vi "メイン.vi"() -> (2 "測定周期/ms":dbl, 3 "値転記用配列":T2[](array[typedef]))   [LabVIEW 2021] (continued)
                          n3108 = Add(x=w5491, y=10) -> (x+y=w5482:i32)
                          n3109 = local read "csv作成表"() -> (w5478:string[][])
                          n3110 = Unbundle By Name(w5489) -> ("実測値(MAX)"=w5485:string, "実測値(MIN)"=w5486:string)
                          n3111 = Replace Array Subset(array=w5478, new element #1=w5485, index (row) #1=w5483, index (col) #1=w5484, new element #2=w5486, index (row) #2=w5483, index (col) #2=w5482) -> (w5480:string[][])
                          n3112 = Select(t=w5480, s=w5490, f=w5478) -> (s? t:f=w5481:string[][])
                          n3113 = local write "csv作成表"(w5481) -> ()
                        }
                        frame 8 {
                          w5501 = 2
                          # "B"
                          # "A"
                          # "csv作成の為表へクラスタ(実測値)書き込み"
                          # "⑤"
                          # "③"
                          # "④"
                          n3114 = local read "メインON/OFF_\n設定 9"() -> (w5512:T1)
                          n3115 = Unbundle By Name(w5512) -> ("使用ON/OFF"=w5508:bool)
                          n3116 = control-ref of="前回値転記用配列"() -> (w5506:refnum<vi>)
                          n3117 = local read "メイン設定_設定 9"() -> (w5513:T2)
                          n3118 = call "メイン_測定値配列_CSV転記サブ.vi"("メイン設定_設定入力"=w5513, "ループ反復数値入力"=w5510, "実測設定項目"=w5511, "使用ON/OFF"=w5508, "前回値転記用配列"=w5506) -> ("ループ反復数値出力"=w5509:i32, "メイン設定_設定出力"=w5507:T2)  [unwired: 5 in]
                          n3119 = local write "メイン設定_設定 9"(w5507) -> ()
                          n3120 = Add(x=10, y=w5509) -> (x+y=w5502:i32)
                          n3121 = Add(x=w5509, y=11) -> (x+y=w5500:i32)
                          n3122 = local read "csv作成表"() -> (w5496:string[][])
                          n3123 = Unbundle By Name(w5507) -> ("実測値(MAX)"=w5503:string, "実測値(MIN)"=w5504:string)
                          n3124 = Replace Array Subset(array=w5496, new element #1=w5503, index (row) #1=w5501, index (col) #1=w5502, new element #2=w5504, index (row) #2=w5501, index (col) #2=w5500) -> (w5498:string[][])
                          n3125 = Select(t=w5498, s=w5508, f=w5496) -> (s? t:f=w5499:string[][])
                          n3126 = local write "csv作成表"(w5499) -> ()
                        }
                        frame 9 {
                          w5519 = 2
                          # "B"
                          # "A"
                          # "csv作成の為表へクラスタ(実測値)書き込み"
                          # "⑤"
                          # "③"
                          # "④"
                          n3127 = local read "メインON/OFF_\n設定 10"() -> (w5530:T1)
                          n3128 = Unbundle By Name(w5530) -> ("使用ON/OFF"=w5526:bool)
                          n3129 = control-ref of="前回値転記用配列"() -> (w5524:refnum<vi>)
                          n3130 = local read "メイン設定_設定 10"() -> (w5531:T2)
                          n3131 = call "メイン_測定値配列_CSV転記サブ.vi"("メイン設定_設定入力"=w5531, "ループ反復数値入力"=w5528, "実測設定項目"=w5529, "使用ON/OFF"=w5526, "前回値転記用配列"=w5524) -> ("ループ反復数値出力"=w5527:i32, "メイン設定_設定出力"=w5525:T2)  [unwired: 5 in]
                          n3132 = local write "メイン設定_設定 10"(w5525) -> ()
                          n3133 = Add(x=11, y=w5527) -> (x+y=w5520:i32)
                          n3134 = Add(x=w5527, y=12) -> (x+y=w5518:i32)
                          n3135 = local read "csv作成表"() -> (w5514:string[][])
                          n3136 = Unbundle By Name(w5525) -> ("実測値(MAX)"=w5521:string, "実測値(MIN)"=w5522:string)
                          n3137 = Replace Array Subset(array=w5514, new element #1=w5521, index (row) #1=w5519, index (col) #1=w5520, new element #2=w5522, index (row) #2=w5519, index (col) #2=w5518) -> (w5516:string[][])
                          n3138 = Select(t=w5516, s=w5526, f=w5514) -> (s? t:f=w5517:string[][])
                          n3139 = local write "csv作成表"(w5517) -> ()
                        }
                        frame 10 {
                          w5537 = 2
                          # "B"
                          # "A"
                          # "csv作成の為表へクラスタ(実測値)書き込み"
                          # "⑤"
                          # "③"
                          # "④"
                          n3140 = local read "メインON/OFF_\n設定 11"() -> (w5548:T1)
                          n3141 = Unbundle By Name(w5548) -> ("使用ON/OFF"=w5544:bool)
                          n3142 = control-ref of="前回値転記用配列"() -> (w5542:refnum<vi>)
                          n3143 = local read "メイン設定_設定 11"() -> (w5549:T2)
                          n3144 = call "メイン_測定値配列_CSV転記サブ.vi"("メイン設定_設定入力"=w5549, "ループ反復数値入力"=w5546, "実測設定項目"=w5547, "使用ON/OFF"=w5544, "前回値転記用配列"=w5542) -> ("ループ反復数値出力"=w5545:i32, "メイン設定_設定出力"=w5543:T2)  [unwired: 5 in]
                          n3145 = local write "メイン設定_設定 11"(w5543) -> ()
                          n3146 = Add(x=12, y=w5545) -> (x+y=w5538:i32)
                          n3147 = Add(x=w5545, y=13) -> (x+y=w5536:i32)
                          n3148 = local read "csv作成表"() -> (w5532:string[][])
                          n3149 = Unbundle By Name(w5543) -> ("実測値(MAX)"=w5539:string, "実測値(MIN)"=w5540:string)
                          n3150 = Replace Array Subset(array=w5532, new element #1=w5539, index (row) #1=w5537, index (col) #1=w5538, new element #2=w5540, index (row) #2=w5537, index (col) #2=w5536) -> (w5534:string[][])
                          n3151 = Select(t=w5534, s=w5544, f=w5532) -> (s? t:f=w5535:string[][])
                          n3152 = local write "csv作成表"(w5535) -> ()
                        }
                        frame 11 {
                          w5555 = 2
                          # "B"
                          # "A"
                          # "csv作成の為表へクラスタ(実測値)書き込み"
                          # "⑤"
                          # "③"
                          # "④"
                          n3153 = local read "メインON/OFF_\n設定 12"() -> (w5566:T1)
                          n3154 = Unbundle By Name(w5566) -> ("使用ON/OFF"=w5562:bool)
                          n3155 = control-ref of="前回値転記用配列"() -> (w5560:refnum<vi>)
                          n3156 = local read "メイン設定_設定 12"() -> (w5567:T2)
                          n3157 = call "メイン_測定値配列_CSV転記サブ.vi"("メイン設定_設定入力"=w5567, "ループ反復数値入力"=w5564, "実測設定項目"=w5565, "使用ON/OFF"=w5562, "前回値転記用配列"=w5560) -> ("ループ反復数値出力"=w5563:i32, "メイン設定_設定出力"=w5561:T2)  [unwired: 5 in]
                          n3158 = local write "メイン設定_設定 12"(w5561) -> ()
                          n3159 = Add(x=13, y=w5563) -> (x+y=w5556:i32)
                          n3160 = Add(x=w5563, y=14) -> (x+y=w5554:i32)
                          n3161 = local read "csv作成表"() -> (w5550:string[][])
                          n3162 = Unbundle By Name(w5561) -> ("実測値(MAX)"=w5557:string, "実測値(MIN)"=w5558:string)
                          n3163 = Replace Array Subset(array=w5550, new element #1=w5557, index (row) #1=w5555, index (col) #1=w5556, new element #2=w5558, index (row) #2=w5555, index (col) #2=w5554) -> (w5552:string[][])
                          n3164 = Select(t=w5552, s=w5562, f=w5550) -> (s? t:f=w5553:string[][])
                          n3165 = local write "csv作成表"(w5553) -> ()
                        }
                      }
                    }
                  }
                }
                n3166 = local write "値転記用配列"(w5324) -> ()
                n3167 = flat-sequence {
                  tunnel: [w5339] -> w5325
                  tunnel: w5324 -> [w5339]
                  frame #0 {
                    w5334 = T9 {"Horizontal"=-51, "Vertical"=504} ("座標 7")
                    n3168 = control-ref of="このVI"() -> (w5335:refnum<vi>)
                    n3169 = property on="ペーン 2" class="Pane"("Origin"=w5334) -> ()  [unwired: 2 in, 2 out]
                    n3170 = property on="ペーン 2" class="Pane"("Origin"=w5334) -> ()  [unwired: 2 in, 2 out]
                    n3171 = control-ref of="このVI"() -> (w5337:refnum<vi>)
                    n3172 = Unbundle(w5334) -> ("Vertical"=w5336:i16)  [unwired: 1 out]
                    n3173 = Unbundle(w5334) -> ("Vertical"=w5338:i16)  [unwired: 1 out]
                    n3174 = call "メイン_装飾移動サブ.vi"("Y軸座標入力"=w5336, "VI入力"=w5335) -> ()  [unwired: 10 in]
                    n3175 = call "メイン_装飾枠移動サブ.vi"("Y軸座標入力"=w5338, "VI入力"=w5337) -> ()  [unwired: 10 in]
                  }
                }
              }
              frame #1 {
                w5569 = T8."Enabled" ("無効")
                # "⑪ボタンの無効解除"
                n3176 = local write "測定新値\nリセット用 8"(TRUE) -> ()
                n3177 = for {
                  N: 12 -> [_]
                  tunnel: w5569 -> [w5572]
                  i -> [w5573]
                  n3178 = case shown="11" w5573 {
                    tunnel: w5572 -> [w5574 w5575 w5576 w5577 w5578 w5579 w5580 w5581 w5582 w5583 w5584 w5585]
                    frame 0, Default {
                      n3179 = property on="メイン測定ボタン_単発 1" class="Bool (指定)"("DisabledEnum"=w5574) -> ()  [unwired: 2 in, 2 out]
                      n3180 = property on="メイン測定ボタン_連続 1" class="Bool (指定)"("DisabledEnum"=w5574) -> ()  [unwired: 2 in, 2 out]
                    }
                    frame 1 {
                      n3181 = property on="メイン測定ボタン_単発 2" class="Bool (指定)"("DisabledEnum"=w5575) -> ()  [unwired: 2 in, 2 out]
                      n3182 = property on="メイン測定ボタン_連続 2" class="Bool (指定)"("DisabledEnum"=w5575) -> ()  [unwired: 2 in, 2 out]
                    }
                    frame 2 {
                      n3183 = property on="メイン測定ボタン_単発 3" class="Bool (指定)"("DisabledEnum"=w5576) -> ()  [unwired: 2 in, 2 out]
                      n3184 = property on="メイン測定ボタン_連続 3" class="Bool (指定)"("DisabledEnum"=w5576) -> ()  [unwired: 2 in, 2 out]
                    }
                    frame 3 {
                      n3185 = property on="メイン測定ボタン_単発 4" class="Bool (指定)"("DisabledEnum"=w5577) -> ()  [unwired: 2 in, 2 out]
                      n3186 = property on="メイン測定ボタン_連続 4" class="Bool (指定)"("DisabledEnum"=w5577) -> ()  [unwired: 2 in, 2 out]
                    }
                    frame 4 {
                      n3187 = property on="メイン測定ボタン_単発 5" class="Bool (指定)"("DisabledEnum"=w5578) -> ()  [unwired: 2 in, 2 out]
                      n3188 = property on="メイン測定ボタン_連続 5" class="Bool (指定)"("DisabledEnum"=w5578) -> ()  [unwired: 2 in, 2 out]
                    }
                    frame 5 {
                      n3189 = property on="メイン測定ボタン_連続 6" class="Bool (指定)"("DisabledEnum"=w5579) -> ()  [unwired: 2 in, 2 out]
                      n3190 = property on="メイン測定ボタン_単発 6" class="Bool (指定)"("DisabledEnum"=w5579) -> ()  [unwired: 2 in, 2 out]
                    }
                    frame 6 {
                      n3191 = property on="メイン測定ボタン_連続 7" class="Bool (指定)"("DisabledEnum"=w5580) -> ()  [unwired: 2 in, 2 out]
                      n3192 = property on="メイン測定ボタン_単発 7" class="Bool (指定)"("DisabledEnum"=w5580) -> ()  [unwired: 2 in, 2 out]
                    }
                    frame 7 {
                      n3193 = property on="メイン測定ボタン_単発 8" class="Bool (指定)"("DisabledEnum"=w5581) -> ()  [unwired: 2 in, 2 out]
                      n3194 = property on="メイン測定ボタン_連続 8" class="Bool (指定)"("DisabledEnum"=w5581) -> ()  [unwired: 2 in, 2 out]
                    }
                    frame 8 {
                      n3195 = property on="メイン測定ボタン_単発 9" class="Bool (指定)"("DisabledEnum"=w5582) -> ()  [unwired: 2 in, 2 out]
                      n3196 = property on="メイン測定ボタン_連続 9" class="Bool (指定)"("DisabledEnum"=w5582) -> ()  [unwired: 2 in, 2 out]
                    }
                    frame 9 {
                      n3197 = property on="メイン測定ボタン_単発 10" class="Bool (指定)"("DisabledEnum"=w5583) -> ()  [unwired: 2 in, 2 out]
                      n3198 = property on="メイン測定ボタン_連続 10" class="Bool (指定)"("DisabledEnum"=w5583) -> ()  [unwired: 2 in, 2 out]
                    }
                    frame 10 {
                      n3199 = property on="メイン測定ボタン_単発 11" class="Bool (指定)"("DisabledEnum"=w5584) -> ()  [unwired: 2 in, 2 out]
                      n3200 = property on="メイン測定ボタン_連続 11" class="Bool (指定)"("DisabledEnum"=w5584) -> ()  [unwired: 2 in, 2 out]
                    }
                    frame 11 {
                      n3201 = property on="メイン測定ボタン_連続 12" class="Bool (指定)"("DisabledEnum"=w5585) -> ()  [unwired: 2 in, 2 out]
                      n3202 = property on="メイン測定ボタン_単発 12" class="Bool (指定)"("DisabledEnum"=w5585) -> ()  [unwired: 2 in, 2 out]
                    }
                  }
                }
                n3203 = property on="TOPページへ" class="Bool"("DisabledEnum"=w5569) -> ()  [unwired: 2 in, 2 out]
                n3204 = property on="保存して終了" class="Bool"("DisabledEnum"=w5569) -> ()  [unwired: 2 in, 2 out]
                n3205 = property on="保存せずに" class="Bool"("DisabledEnum"=w5569) -> ()  [unwired: 2 in, 2 out]
              }
            }
          }
          frame True {
          }
        }
      }
      frame "測定9" {
        # "⑦"
        # "項目別のボタンで測定を行う為、項目分必要"
        n3206 = local read "測定旧値 9"() -> (w5589:bool)
        n3207 = case shown="FALSE" w5589 {
          tunnel: w5587 -> [w5592 w5855]
          tunnel: [w5591 w5855] -> w5588
          frame False {
            n3208 = flat-sequence {
              tunnel: w5592 -> [w5602]
              tunnel: [w5594] -> w5590
              tunnel: [w5840] -> w5591
              tunnel: w5590 -> [w5840]
              frame #0 {
                # "※複製コピー時変更する項目\n①②\nローカル変数\n\n入れ子のケースストラクチャ\"2\"を複製\n\n0～数だけ変更する\n③④⑤\nローカル変数\n\n※AB\n行番号の変更をする必要がある\n\n--------------------------------\nこの後イベントストラクチャ複製する\n--------------------------------\nイベントストラクチャ複製後\n\n⑦⑧\nローカル変数\n⑨\n装飾体の位置設定\n-51は固定\n前ケースの数値+72\n⑩\n測定新値リセット用\nのボタンが複製されているので、\nフロントパネルを整理する\n⑪\nプロパティノード\nボタンの無効解除クリア以外全てのボタン対象"
                # "実測完了の簡易疑似コード\n\n1)測定モードが単発・連続、多点かで転記する配列を変える\n2)値転記用配列へ転記\n\nここからゲージ分を繰り返す必要がある\n\n3)配列0を取り出す\n4)配列0のポートNoを取り出す\n5)メイン測定_設定配列(測定1の対象配列)のポートNoと比較\n6)同じだったら処理をする。違ったら何もしない\n7)同じだったら配列0のメインON/OFF_設定1の使用ON/OFFがTrueかFalseか\nFlaseだったら前回値転記用配列から前回の値をメイン設定_設定へ転記\nTrueだったらメイン設定_設定の測定モードから\n0単発、1連続、3多点\nの処理を行う\n8)測定値をメイン設定_設定へ転記したら、前回転記用配列へ転記する"
                # "⑨"
                # "⑧"
                # "②"
                # "グループNO(表示上はポートNo)が同じだったら値を転記する\n\n測定した配列のグループNOと値転記用配列の他の指標グループNOを比較する\n＝だったら、対象の配列のON/OFFボタンがTrueか確認し、\nTrueだったら、測定モードによって、値かMAX、MINの数値を転記する\n\nグループNOが同じでなければ、転記しない(何もしない)"
                # "まず値転記用配列に測定の値を転記"
                # "実測定画面vi動作"
                n3209 = local read "メイン設定_設定 9"() -> (w5597:T2)
                n3210 = local read "測定新値 9"() -> (→"測定新値\nリセット用 9":bool)
                n3211 = local read "測定周期/ms"() -> (w5595:dbl)
                n3212 = Unbundle By Name(w5597) -> ("測定モード"=w5598:u16)
                n3213 = call "実測定画面.vi"("実測設定項目配列_\nメインからの転記"=w5602, "測定周期/ms_制御器"=w5595) -> ("実測設定項目配列_\nゲージIOへ転記用"=w5600:T2[], "実測設定項目配列_\n多点測定メイン転記用"=w5599:T2[])  [unwired: 11 in, 1 out]
                n3214 = case shown="1" w5598 {
                  tunnel: w5600 -> [w5609 w5610 _]
                  tunnel: [w5609 w5610 w5611] -> w5593
                  tunnel: w5599 -> [_ _ w5611]
                  frame 0, Default {
                  }
                  frame 1 {
                  }
                  frame 2 {
                  }
                }
                n3215 = for {
                  N: 32 -> [_]
                  tunnel: w5593 -> [w5618]
                  i -> [w5613]
                  # "①"
                  # "※複製コピーはこのケースで行う"
                  # "32回分"
                  # "比較する固定GNO"
                  n3216 = local read "メイン設定_設定 9"() -> (w5612:T2)
                  n3217 = Index Array(array=w5618, index=w5613) -> (element=w5617:T2)
                  n3218 = Unbundle By Name(w5612) -> ("ポートNo."=w5616:dbl)
                  n3219 = Unbundle By Name(w5617) -> ("ポートNo."=w5615:dbl)
                  n3220 = Equal?(x=w5616, y=w5615) -> (x = y?=w5614:bool)
                  n3221 = case shown="TRUE" w5614 {
                    tunnel: w5617 -> [_ w5620]
                    tunnel: w5613 -> [_ w5619]
                    frame False {
                    }
                    frame True {
                      n3222 = case shown="0, デフォルト" w5619 {
                        tunnel: w5620 -> [w5636 w5654 w5672 w5690 w5708 w5726 w5744 w5762 w5780 w5798 w5816 w5834]
                        tunnel: w5619 -> [w5635 w5653 w5671 w5689 w5707 w5725 w5743 w5761 w5779 w5797 w5815 w5833]
                        frame 0, Default {
                          w5626 = 2
                          # "B"
                          # "A"
                          # "csv作成の為表へクラスタ(実測値)書き込み"
                          # "⑤"
                          # "③"
                          # "④"
                          n3223 = local read "メインON/OFF_\n設定 1"() -> (w5637:T1)
                          n3224 = Unbundle By Name(w5637) -> ("使用ON/OFF"=w5633:bool)
                          n3225 = control-ref of="前回値転記用配列"() -> (w5631:refnum<vi>)
                          n3226 = local read "メイン設定_設定 1"() -> (w5638:T2)
                          n3227 = call "メイン_測定値配列_CSV転記サブ.vi"("メイン設定_設定入力"=w5638, "ループ反復数値入力"=w5635, "実測設定項目"=w5636, "使用ON/OFF"=w5633, "前回値転記用配列"=w5631) -> ("ループ反復数値出力"=w5634:i32, "メイン設定_設定出力"=w5632:T2)  [unwired: 5 in]
                          n3228 = local write "メイン設定_設定 1"(w5632) -> ()
                          n3229 = Add(x=2, y=w5634) -> (x+y=w5627:i32)
                          n3230 = Add(x=w5634, y=3) -> (x+y=w5625:i32)
                          n3231 = local read "csv作成表"() -> (w5621:string[][])
                          n3232 = Unbundle By Name(w5632) -> ("実測値(MAX)"=w5628:string, "実測値(MIN)"=w5629:string)
                          n3233 = Replace Array Subset(array=w5621, new element #1=w5628, index (row) #1=w5626, index (col) #1=w5627, new element #2=w5629, index (row) #2=w5626, index (col) #2=w5625) -> (w5623:string[][])
                          n3234 = Select(t=w5623, s=w5633, f=w5621) -> (s? t:f=w5624:string[][])
                          n3235 = local write "csv作成表"(w5624) -> ()
                        }
                        frame 1 {
                          w5644 = 2
                          # "B"
                          # "A"
                          # "csv作成の為表へクラスタ(実測値)書き込み"
                          # "⑤"
                          # "③"
                          # "④"
                          n3236 = local read "メインON/OFF_\n設定 2"() -> (w5655:T1)
                          n3237 = Unbundle By Name(w5655) -> ("使用ON/OFF"=w5651:bool)
                          n3238 = control-ref of="前回値転記用配列"() -> (w5649:refnum<vi>)
                          n3239 = local read "メイン設定_設定 2"() -> (w5656:T2)
                          n3240 = call "メイン_測定値配列_CSV転記サブ.vi"("メイン設定_設定入力"=w5656, "ループ反復数値入力"=w5653, "実測設定項目"=w5654, "使用ON/OFF"=w5651, "前回値転記用配列"=w5649) -> ("ループ反復数値出力"=w5652:i32, "メイン設定_設定出力"=w5650:T2)  [unwired: 5 in]
                          n3241 = local write "メイン設定_設定 2"(w5650) -> ()
                          n3242 = Add(x=3, y=w5652) -> (x+y=w5645:i32)
                          n3243 = Add(x=w5652, y=4) -> (x+y=w5643:i32)
                          n3244 = local read "csv作成表"() -> (w5639:string[][])
                          n3245 = Unbundle By Name(w5650) -> ("実測値(MAX)"=w5646:string, "実測値(MIN)"=w5647:string)
                          n3246 = Replace Array Subset(array=w5639, new element #1=w5646, index (row) #1=w5644, index (col) #1=w5645, new element #2=w5647, index (row) #2=w5644, index (col) #2=w5643) -> (w5641:string[][])
                          n3247 = Select(t=w5641, s=w5651, f=w5639) -> (s? t:f=w5642:string[][])
                          n3248 = local write "csv作成表"(w5642) -> ()
                        }
                        frame 2 {
                          w5662 = 2
                          # "B"
                          # "A"
                          # "csv作成の為表へクラスタ(実測値)書き込み"
                          # "⑤"
                          # "③"
                          # "④"
                          n3249 = local read "メインON/OFF_\n設定 3"() -> (w5673:T1)
                          n3250 = Unbundle By Name(w5673) -> ("使用ON/OFF"=w5669:bool)
                          n3251 = control-ref of="前回値転記用配列"() -> (w5667:refnum<vi>)
                          n3252 = local read "メイン設定_設定 3"() -> (w5674:T2)
                          n3253 = call "メイン_測定値配列_CSV転記サブ.vi"("メイン設定_設定入力"=w5674, "ループ反復数値入力"=w5671, "実測設定項目"=w5672, "使用ON/OFF"=w5669, "前回値転記用配列"=w5667) -> ("ループ反復数値出力"=w5670:i32, "メイン設定_設定出力"=w5668:T2)  [unwired: 5 in]
                          n3254 = local write "メイン設定_設定 3"(w5668) -> ()
                          n3255 = Add(x=4, y=w5670) -> (x+y=w5663:i32)
                          n3256 = Add(x=w5670, y=5) -> (x+y=w5661:i32)
                          n3257 = local read "csv作成表"() -> (w5657:string[][])
                          n3258 = Unbundle By Name(w5668) -> ("実測値(MAX)"=w5664:string, "実測値(MIN)"=w5665:string)
                          n3259 = Replace Array Subset(array=w5657, new element #1=w5664, index (row) #1=w5662, index (col) #1=w5663, new element #2=w5665, index (row) #2=w5662, index (col) #2=w5661) -> (w5659:string[][])
                          n3260 = Select(t=w5659, s=w5669, f=w5657) -> (s? t:f=w5660:string[][])
                          n3261 = local write "csv作成表"(w5660) -> ()
                        }
                        frame 3 {
                          w5680 = 2
                          # "B"
                          # "A"
                          # "csv作成の為表へクラスタ(実測値)書き込み"
                          # "⑤"
                          # "③"
                          # "④"
                          n3262 = local read "メインON/OFF_\n設定 4"() -> (w5691:T1)
                          n3263 = Unbundle By Name(w5691) -> ("使用ON/OFF"=w5687:bool)
                          n3264 = control-ref of="前回値転記用配列"() -> (w5685:refnum<vi>)
                          n3265 = local read "メイン設定_設定 4"() -> (w5692:T2)
                          n3266 = call "メイン_測定値配列_CSV転記サブ.vi"("メイン設定_設定入力"=w5692, "ループ反復数値入力"=w5689, "実測設定項目"=w5690, "使用ON/OFF"=w5687, "前回値転記用配列"=w5685) -> ("ループ反復数値出力"=w5688:i32, "メイン設定_設定出力"=w5686:T2)  [unwired: 5 in]
                          n3267 = local write "メイン設定_設定 4"(w5686) -> ()
                          n3268 = Add(x=5, y=w5688) -> (x+y=w5681:i32)
                          n3269 = Add(x=w5688, y=6) -> (x+y=w5679:i32)
                          n3270 = local read "csv作成表"() -> (w5675:string[][])
                          n3271 = Unbundle By Name(w5686) -> ("実測値(MAX)"=w5682:string, "実測値(MIN)"=w5683:string)
                          n3272 = Replace Array Subset(array=w5675, new element #1=w5682, index (row) #1=w5680, index (col) #1=w5681, new element #2=w5683, index (row) #2=w5680, index (col) #2=w5679) -> (w5677:string[][])
                          n3273 = Select(t=w5677, s=w5687, f=w5675) -> (s? t:f=w5678:string[][])
                          n3274 = local write "csv作成表"(w5678) -> ()
                        }
                        frame 4 {
                          w5698 = 2
                          # "B"
                          # "A"
                          # "csv作成の為表へクラスタ(実測値)書き込み"
                          # "⑤"
                          # "③"
                          # "④"
                          n3275 = local read "メインON/OFF_\n設定 5"() -> (w5709:T1)
                          n3276 = Unbundle By Name(w5709) -> ("使用ON/OFF"=w5705:bool)
                          n3277 = control-ref of="前回値転記用配列"() -> (w5703:refnum<vi>)
                          n3278 = local read "メイン設定_設定 5"() -> (w5710:T2)
                          n3279 = call "メイン_測定値配列_CSV転記サブ.vi"("メイン設定_設定入力"=w5710, "ループ反復数値入力"=w5707, "実測設定項目"=w5708, "使用ON/OFF"=w5705, "前回値転記用配列"=w5703) -> ("ループ反復数値出力"=w5706:i32, "メイン設定_設定出力"=w5704:T2)  [unwired: 5 in]
                          n3280 = local write "メイン設定_設定 5"(w5704) -> ()
                          n3281 = Add(x=6, y=w5706) -> (x+y=w5699:i32)
                          n3282 = Add(x=w5706, y=7) -> (x+y=w5697:i32)
                          n3283 = local read "csv作成表"() -> (w5693:string[][])
                          n3284 = Unbundle By Name(w5704) -> ("実測値(MAX)"=w5700:string, "実測値(MIN)"=w5701:string)
                          n3285 = Replace Array Subset(array=w5693, new element #1=w5700, index (row) #1=w5698, index (col) #1=w5699, new element #2=w5701, index (row) #2=w5698, index (col) #2=w5697) -> (w5695:string[][])
                          n3286 = Select(t=w5695, s=w5705, f=w5693) -> (s? t:f=w5696:string[][])
                          n3287 = local write "csv作成表"(w5696) -> ()
                        }
                        frame 5 {
                          w5716 = 2
                          # "B"
                          # "A"
                          # "csv作成の為表へクラスタ(実測値)書き込み"
                          # "⑤"
                          # "③"
                          # "④"
                          n3288 = local read "メインON/OFF_\n設定 6"() -> (w5727:T1)
                          n3289 = Unbundle By Name(w5727) -> ("使用ON/OFF"=w5723:bool)
                          n3290 = control-ref of="前回値転記用配列"() -> (w5721:refnum<vi>)
                          n3291 = local read "メイン設定_設定 6"() -> (w5728:T2)
                          n3292 = call "メイン_測定値配列_CSV転記サブ.vi"("メイン設定_設定入力"=w5728, "ループ反復数値入力"=w5725, "実測設定項目"=w5726, "使用ON/OFF"=w5723, "前回値転記用配列"=w5721) -> ("ループ反復数値出力"=w5724:i32, "メイン設定_設定出力"=w5722:T2)  [unwired: 5 in]
                          n3293 = local write "メイン設定_設定 6"(w5722) -> ()
                          n3294 = Add(x=7, y=w5724) -> (x+y=w5717:i32)
                          n3295 = Add(x=w5724, y=8) -> (x+y=w5715:i32)
                          n3296 = local read "csv作成表"() -> (w5711:string[][])
                          n3297 = Unbundle By Name(w5722) -> ("実測値(MAX)"=w5718:string, "実測値(MIN)"=w5719:string)
                          n3298 = Replace Array Subset(array=w5711, new element #1=w5718, index (row) #1=w5716, index (col) #1=w5717, new element #2=w5719, index (row) #2=w5716, index (col) #2=w5715) -> (w5713:string[][])
                          n3299 = Select(t=w5713, s=w5723, f=w5711) -> (s? t:f=w5714:string[][])
                          n3300 = local write "csv作成表"(w5714) -> ()
                        }
                        frame 6 {
                          w5734 = 2
                          # "B"
                          # "A"
                          # "csv作成の為表へクラスタ(実測値)書き込み"
                          # "⑤"
                          # "③"
                          # "④"
                          n3301 = local read "メインON/OFF_\n設定 7"() -> (w5745:T1)
                          n3302 = Unbundle By Name(w5745) -> ("使用ON/OFF"=w5741:bool)
                          n3303 = control-ref of="前回値転記用配列"() -> (w5739:refnum<vi>)
                          n3304 = local read "メイン設定_設定 7"() -> (w5746:T2)
                          n3305 = call "メイン_測定値配列_CSV転記サブ.vi"("メイン設定_設定入力"=w5746, "ループ反復数値入力"=w5743, "実測設定項目"=w5744, "使用ON/OFF"=w5741, "前回値転記用配列"=w5739) -> ("ループ反復数値出力"=w5742:i32, "メイン設定_設定出力"=w5740:T2)  [unwired: 5 in]
                          n3306 = local write "メイン設定_設定 7"(w5740) -> ()
                          n3307 = Add(x=8, y=w5742) -> (x+y=w5735:i32)
                          n3308 = Add(x=w5742, y=9) -> (x+y=w5733:i32)
                          n3309 = local read "csv作成表"() -> (w5729:string[][])
                          n3310 = Unbundle By Name(w5740) -> ("実測値(MAX)"=w5736:string, "実測値(MIN)"=w5737:string)
                          n3311 = Replace Array Subset(array=w5729, new element #1=w5736, index (row) #1=w5734, index (col) #1=w5735, new element #2=w5737, index (row) #2=w5734, index (col) #2=w5733) -> (w5731:string[][])
                          n3312 = Select(t=w5731, s=w5741, f=w5729) -> (s? t:f=w5732:string[][])
                          n3313 = local write "csv作成表"(w5732) -> ()
                        }
                        frame 7 {
                          w5752 = 2
                          # "B"
                          # "A"
                          # "csv作成の為表へクラスタ(実測値)書き込み"
                          # "⑤"
                          # "③"
                          # "④"
                          n3314 = local read "メインON/OFF_\n設定 8"() -> (w5763:T1)
                          n3315 = Unbundle By Name(w5763) -> ("使用ON/OFF"=w5759:bool)
                          n3316 = control-ref of="前回値転記用配列"() -> (w5757:refnum<vi>)
                          n3317 = local read "メイン設定_設定 8"() -> (w5764:T2)
                          n3318 = call "メイン_測定値配列_CSV転記サブ.vi"("メイン設定_設定入力"=w5764, "ループ反復数値入力"=w5761, "実測設定項目"=w5762, "使用ON/OFF"=w5759, "前回値転記用配列"=w5757) -> ("ループ反復数値出力"=w5760:i32, "メイン設定_設定出力"=w5758:T2)  [unwired: 5 in]
                          n3319 = local write "メイン設定_設定 8"(w5758) -> ()
                          n3320 = Add(x=9, y=w5760) -> (x+y=w5753:i32)
                          n3321 = Add(x=w5760, y=10) -> (x+y=w5751:i32)
                          n3322 = local read "csv作成表"() -> (w5747:string[][])
                          n3323 = Unbundle By Name(w5758) -> ("実測値(MAX)"=w5754:string, "実測値(MIN)"=w5755:string)
                          n3324 = Replace Array Subset(array=w5747, new element #1=w5754, index (row) #1=w5752, index (col) #1=w5753, new element #2=w5755, index (row) #2=w5752, index (col) #2=w5751) -> (w5749:string[][])
                          n3325 = Select(t=w5749, s=w5759, f=w5747) -> (s? t:f=w5750:string[][])
                          n3326 = local write "csv作成表"(w5750) -> ()
                        }
                        frame 8 {
                          w5770 = 2
                          # "B"
                          # "A"
                          # "csv作成の為表へクラスタ(実測値)書き込み"
                          # "⑤"
                          # "③"
                          # "④"
                          n3327 = local read "メインON/OFF_\n設定 9"() -> (w5781:T1)
                          n3328 = Unbundle By Name(w5781) -> ("使用ON/OFF"=w5777:bool)
                          n3329 = control-ref of="前回値転記用配列"() -> (w5775:refnum<vi>)
                          n3330 = local read "メイン設定_設定 9"() -> (w5782:T2)
                          n3331 = call "メイン_測定値配列_CSV転記サブ.vi"("メイン設定_設定入力"=w5782, "ループ反復数値入力"=w5779, "実測設定項目"=w5780, "使用ON/OFF"=w5777, "前回値転記用配列"=w5775) -> ("ループ反復数値出力"=w5778:i32, "メイン設定_設定出力"=w5776:T2)  [unwired: 5 in]
                          n3332 = local write "メイン設定_設定 9"(w5776) -> ()
                          n3333 = Add(x=10, y=w5778) -> (x+y=w5771:i32)
                          n3334 = Add(x=w5778, y=11) -> (x+y=w5769:i32)
                          n3335 = local read "csv作成表"() -> (w5765:string[][])
                          n3336 = Unbundle By Name(w5776) -> ("実測値(MAX)"=w5772:string, "実測値(MIN)"=w5773:string)
                          n3337 = Replace Array Subset(array=w5765, new element #1=w5772, index (row) #1=w5770, index (col) #1=w5771, new element #2=w5773, index (row) #2=w5770, index (col) #2=w5769) -> (w5767:string[][])
                          n3338 = Select(t=w5767, s=w5777, f=w5765) -> (s? t:f=w5768:string[][])
                          n3339 = local write "csv作成表"(w5768) -> ()
                        }
                        frame 9 {
                          w5788 = 2
                          # "B"
                          # "A"
                          # "csv作成の為表へクラスタ(実測値)書き込み"
                          # "⑤"
                          # "③"
                          # "④"
                          n3340 = local read "メインON/OFF_\n設定 10"() -> (w5799:T1)
                          n3341 = Unbundle By Name(w5799) -> ("使用ON/OFF"=w5795:bool)
                          n3342 = control-ref of="前回値転記用配列"() -> (w5793:refnum<vi>)
                          n3343 = local read "メイン設定_設定 10"() -> (w5800:T2)
                          n3344 = call "メイン_測定値配列_CSV転記サブ.vi"("メイン設定_設定入力"=w5800, "ループ反復数値入力"=w5797, "実測設定項目"=w5798, "使用ON/OFF"=w5795, "前回値転記用配列"=w5793) -> ("ループ反復数値出力"=w5796:i32, "メイン設定_設定出力"=w5794:T2)  [unwired: 5 in]
                          n3345 = local write "メイン設定_設定 10"(w5794) -> ()
                          n3346 = Add(x=11, y=w5796) -> (x+y=w5789:i32)
                          n3347 = Add(x=w5796, y=12) -> (x+y=w5787:i32)
                          n3348 = local read "csv作成表"() -> (w5783:string[][])
                          n3349 = Unbundle By Name(w5794) -> ("実測値(MAX)"=w5790:string, "実測値(MIN)"=w5791:string)
                          n3350 = Replace Array Subset(array=w5783, new element #1=w5790, index (row) #1=w5788, index (col) #1=w5789, new element #2=w5791, index (row) #2=w5788, index (col) #2=w5787) -> (w5785:string[][])
                          n3351 = Select(t=w5785, s=w5795, f=w5783) -> (s? t:f=w5786:string[][])
                          n3352 = local write "csv作成表"(w5786) -> ()
                        }
                        frame 10 {
                          w5806 = 2
                          # "B"
                          # "A"
                          # "csv作成の為表へクラスタ(実測値)書き込み"
                          # "⑤"
                          # "③"
                          # "④"
                          n3353 = local read "メインON/OFF_\n設定 11"() -> (w5817:T1)
                          n3354 = Unbundle By Name(w5817) -> ("使用ON/OFF"=w5813:bool)
                          n3355 = control-ref of="前回値転記用配列"() -> (w5811:refnum<vi>)
                          n3356 = local read "メイン設定_設定 11"() -> (w5818:T2)
                          n3357 = call "メイン_測定値配列_CSV転記サブ.vi"("メイン設定_設定入力"=w5818, "ループ反復数値入力"=w5815, "実測設定項目"=w5816, "使用ON/OFF"=w5813, "前回値転記用配列"=w5811) -> ("ループ反復数値出力"=w5814:i32, "メイン設定_設定出力"=w5812:T2)  [unwired: 5 in]
                          n3358 = local write "メイン設定_設定 11"(w5812) -> ()
                          n3359 = Add(x=12, y=w5814) -> (x+y=w5807:i32)
                          n3360 = Add(x=w5814, y=13) -> (x+y=w5805:i32)
                          n3361 = local read "csv作成表"() -> (w5801:string[][])
                          n3362 = Unbundle By Name(w5812) -> ("実測値(MAX)"=w5808:string, "実測値(MIN)"=w5809:string)
                          n3363 = Replace Array Subset(array=w5801, new element #1=w5808, index (row) #1=w5806, index (col) #1=w5807, new element #2=w5809, index (row) #2=w5806, index (col) #2=w5805) -> (w5803:string[][])
                          n3364 = Select(t=w5803, s=w5813, f=w5801) -> (s? t:f=w5804:string[][])
                          n3365 = local write "csv作成表"(w5804) -> ()
                        }
                        frame 11 {
                          w5824 = 2
                          # "B"
                          # "A"
                          # "csv作成の為表へクラスタ(実測値)書き込み"
                          # "⑤"
                          # "③"
                          # "④"
                          n3366 = local read "メインON/OFF_\n設定 12"() -> (w5835:T1)
                          n3367 = Unbundle By Name(w5835) -> ("使用ON/OFF"=w5831:bool)
                          n3368 = control-ref of="前回値転記用配列"() -> (w5829:refnum<vi>)
                          n3369 = local read "メイン設定_設定 12"() -> (w5836:T2)
                          n3370 = call "メイン_測定値配列_CSV転記サブ.vi"("メイン設定_設定入力"=w5836, "ループ反復数値入力"=w5833, "実測設定項目"=w5834, "使用ON/OFF"=w5831, "前回値転記用配列"=w5829) -> ("ループ反復数値出力"=w5832:i32, "メイン設定_設定出力"=w5830:T2)  [unwired: 5 in]
                          n3371 = local write "メイン設定_設定 12"(w5830) -> ()
                          n3372 = Add(x=13, y=w5832) -> (x+y=w5825:i32)
                          n3373 = Add(x=w5832, y=14) -> (x+y=w5823:i32)
                          n3374 = local read "csv作成表"() -> (w5819:string[][])
                          n3375 = Unbundle By Name(w5830) -> ("実測値(MAX)"=w5826:string, "実測値(MIN)"=w5827:string)
                          n3376 = Replace Array Subset(array=w5819, new element #1=w5826, index (row) #1=w5824, index (col) #1=w5825, new element #2=w5827, index (row) #2=w5824, index (col) #2=w5823) -> (w5821:string[][])
                          n3377 = Select(t=w5821, s=w5831, f=w5819) -> (s? t:f=w5822:string[][])
                          n3378 = local write "csv作成表"(w5822) -> ()
                        }
                      }
                    }
                  }
                }
                n3379 = local write "値転記用配列"(w5593) -> ()
                n3380 = flat-sequence {
                  tunnel: [w5608] -> w5594
                  tunnel: w5593 -> [w5608]
                  frame #0 {
                    w5603 = T9 {"Horizontal"=-51, "Vertical"=576} ("座標 8")
                    n3381 = control-ref of="このVI"() -> (w5604:refnum<vi>)
                    n3382 = property on="ペーン 2" class="Pane"("Origin"=w5603) -> ()  [unwired: 2 in, 2 out]
                    n3383 = property on="ペーン 2" class="Pane"("Origin"=w5603) -> ()  [unwired: 2 in, 2 out]
                    n3384 = control-ref of="このVI"() -> (w5606:refnum<vi>)
                    n3385 = Unbundle(w5603) -> ("Vertical"=w5605:i16)  [unwired: 1 out]
                    n3386 = Unbundle(w5603) -> ("Vertical"=w5607:i16)  [unwired: 1 out]
                    n3387 = call "メイン_装飾移動サブ.vi"("Y軸座標入力"=w5605, "VI入力"=w5604) -> ()  [unwired: 10 in]
                    n3388 = call "メイン_装飾枠移動サブ.vi"("Y軸座標入力"=w5607, "VI入力"=w5606) -> ()  [unwired: 10 in]
                  }
                }
              }
              frame #1 {
                w5838 = T8."Enabled" ("無効")
                # "⑪ボタンの無効解除"
                n3389 = local write "測定新値\nリセット用 9"(TRUE) -> ()
                n3390 = for {
                  N: 12 -> [_]
                  tunnel: w5838 -> [w5841]
                  i -> [w5842]
                  n3391 = case shown="11" w5842 {
                    tunnel: w5841 -> [w5843 w5844 w5845 w5846 w5847 w5848 w5849 w5850 w5851 w5852 w5853 w5854]
                    frame 0, Default {
                      n3392 = property on="メイン測定ボタン_単発 1" class="Bool (指定)"("DisabledEnum"=w5843) -> ()  [unwired: 2 in, 2 out]
                      n3393 = property on="メイン測定ボタン_連続 1" class="Bool (指定)"("DisabledEnum"=w5843) -> ()  [unwired: 2 in, 2 out]
                    }
                    frame 1 {
                      n3394 = property on="メイン測定ボタン_単発 2" class="Bool (指定)"("DisabledEnum"=w5844) -> ()  [unwired: 2 in, 2 out]
                      n3395 = property on="メイン測定ボタン_連続 2" class="Bool (指定)"("DisabledEnum"=w5844) -> ()  [unwired: 2 in, 2 out]
                    }
                    frame 2 {
                      n3396 = property on="メイン測定ボタン_単発 3" class="Bool (指定)"("DisabledEnum"=w5845) -> ()  [unwired: 2 in, 2 out]
                      n3397 = property on="メイン測定ボタン_連続 3" class="Bool (指定)"("DisabledEnum"=w5845) -> ()  [unwired: 2 in, 2 out]
                    }
                    frame 3 {
                      n3398 = property on="メイン測定ボタン_単発 4" class="Bool (指定)"("DisabledEnum"=w5846) -> ()  [unwired: 2 in, 2 out]
                      n3399 = property on="メイン測定ボタン_連続 4" class="Bool (指定)"("DisabledEnum"=w5846) -> ()  [unwired: 2 in, 2 out]
                    }
                    frame 4 {
                      n3400 = property on="メイン測定ボタン_単発 5" class="Bool (指定)"("DisabledEnum"=w5847) -> ()  [unwired: 2 in, 2 out]
                      n3401 = property on="メイン測定ボタン_連続 5" class="Bool (指定)"("DisabledEnum"=w5847) -> ()  [unwired: 2 in, 2 out]
                    }
                    frame 5 {
                      n3402 = property on="メイン測定ボタン_連続 6" class="Bool (指定)"("DisabledEnum"=w5848) -> ()  [unwired: 2 in, 2 out]
                      n3403 = property on="メイン測定ボタン_単発 6" class="Bool (指定)"("DisabledEnum"=w5848) -> ()  [unwired: 2 in, 2 out]
                    }
                    frame 6 {
                      n3404 = property on="メイン測定ボタン_連続 7" class="Bool (指定)"("DisabledEnum"=w5849) -> ()  [unwired: 2 in, 2 out]
                      n3405 = property on="メイン測定ボタン_単発 7" class="Bool (指定)"("DisabledEnum"=w5849) -> ()  [unwired: 2 in, 2 out]
                    }
                    frame 7 {
                      n3406 = property on="メイン測定ボタン_単発 8" class="Bool (指定)"("DisabledEnum"=w5850) -> ()  [unwired: 2 in, 2 out]
                      n3407 = property on="メイン測定ボタン_連続 8" class="Bool (指定)"("DisabledEnum"=w5850) -> ()  [unwired: 2 in, 2 out]
                    }
                    frame 8 {
                      n3408 = property on="メイン測定ボタン_単発 9" class="Bool (指定)"("DisabledEnum"=w5851) -> ()  [unwired: 2 in, 2 out]
                      n3409 = property on="メイン測定ボタン_連続 9" class="Bool (指定)"("DisabledEnum"=w5851) -> ()  [unwired: 2 in, 2 out]
                    }
                    frame 9 {
                      n3410 = property on="メイン測定ボタン_単発 10" class="Bool (指定)"("DisabledEnum"=w5852) -> ()  [unwired: 2 in, 2 out]
                      n3411 = property on="メイン測定ボタン_連続 10" class="Bool (指定)"("DisabledEnum"=w5852) -> ()  [unwired: 2 in, 2 out]
                    }
                    frame 10 {
                      n3412 = property on="メイン測定ボタン_単発 11" class="Bool (指定)"("DisabledEnum"=w5853) -> ()  [unwired: 2 in, 2 out]
                      n3413 = property on="メイン測定ボタン_連続 11" class="Bool (指定)"("DisabledEnum"=w5853) -> ()  [unwired: 2 in, 2 out]
                    }
                    frame 11 {
                      n3414 = property on="メイン測定ボタン_連続 12" class="Bool (指定)"("DisabledEnum"=w5854) -> ()  [unwired: 2 in, 2 out]
                      n3415 = property on="メイン測定ボタン_単発 12" class="Bool (指定)"("DisabledEnum"=w5854) -> ()  [unwired: 2 in, 2 out]
                    }
                  }
                }
                n3416 = property on="TOPページへ" class="Bool"("DisabledEnum"=w5838) -> ()  [unwired: 2 in, 2 out]
                n3417 = property on="保存して終了" class="Bool"("DisabledEnum"=w5838) -> ()  [unwired: 2 in, 2 out]
                n3418 = property on="保存せずに" class="Bool"("DisabledEnum"=w5838) -> ()  [unwired: 2 in, 2 out]
              }
            }
          }
          frame True {
          }
        }
      }
      frame "測定10" {
        # "⑦"
        # "項目別のボタンで測定を行う為、項目分必要"
        n3419 = local read "測定旧値 10"() -> (w5858:bool)
        n3420 = case shown="FALSE" w5858 {
          tunnel: w5856 -> [w5861 w6124]
          tunnel: [w5860 w6124] -> w5857
          frame False {
            n3421 = flat-sequence {
              tunnel: w5861 -> [w5871]
              tunnel: [w5863] -> w5859
              tunnel: [w6109] -> w5860
              tunnel: w5859 -> [w6109]
              frame #0 {
                # "※複製コピー時変更する項目\n①②\nローカル変数\n\n入れ子のケースストラクチャ\"2\"を複製\n\n0～数だけ変更する\n③④⑤\nローカル変数\n\n※AB\n行番号の変更をする必要がある\n\n--------------------------------\nこの後イベントストラクチャ複製する\n--------------------------------\nイベントストラクチャ複製後\n\n⑦⑧\nローカル変数\n⑨\n装飾体の位置設定\n-51は固定\n前ケースの数値+72\n⑩\n測定新値リセット用\nのボタンが複製されているので、\nフロントパネルを整理する\n⑪\nプロパティノード\nボタンの無効解除クリア以外全てのボタン対象"
                # "実測完了の簡易疑似コード\n\n1)測定モードが単発・連続、多点かで転記する配列を変える\n2)値転記用配列へ転記\n\nここからゲージ分を繰り返す必要がある\n\n3)配列0を取り出す\n4)配列0のポートNoを取り出す\n5)メイン測定_設定配列(測定1の対象配列)のポートNoと比較\n6)同じだったら処理をする。違ったら何もしない\n7)同じだったら配列0のメインON/OFF_設定1の使用ON/OFFがTrueかFalseか\nFlaseだったら前回値転記用配列から前回の値をメイン設定_設定へ転記\nTrueだったらメイン設定_設定の測定モードから\n0単発、1連続、3多点\nの処理を行う\n8)測定値をメイン設定_設定へ転記したら、前回転記用配列へ転記する"
                # "⑨"
                # "⑧"
                # "②"
                # "グループNO(表示上はポートNo)が同じだったら値を転記する\n\n測定した配列のグループNOと値転記用配列の他の指標グループNOを比較する\n＝だったら、対象の配列のON/OFFボタンがTrueか確認し、\nTrueだったら、測定モードによって、値かMAX、MINの数値を転記する\n\nグループNOが同じでなければ、転記しない(何もしない)"
                # "まず値転記用配列に測定の値を転記"
                # "実測定画面vi動作"
                n3422 = local read "メイン設定_設定 10"() -> (w5866:T2)
                n3423 = local read "測定新値 10"() -> (→"測定新値\nリセット用 10":bool)
                n3424 = local read "測定周期/ms"() -> (w5864:dbl)
                n3425 = Unbundle By Name(w5866) -> ("測定モード"=w5867:u16)
                n3426 = call "実測定画面.vi"("実測設定項目配列_\nメインからの転記"=w5871, "測定周期/ms_制御器"=w5864) -> ("実測設定項目配列_\nゲージIOへ転記用"=w5869:T2[], "実測設定項目配列_\n多点測定メイン転記用"=w5868:T2[])  [unwired: 11 in, 1 out]
                n3427 = case shown="1" w5867 {
                  tunnel: w5869 -> [w5878 w5879 _]
                  tunnel: [w5878 w5879 w5880] -> w5862
                  tunnel: w5868 -> [_ _ w5880]
                  frame 0, Default {
                  }
                  frame 1 {
                  }
                  frame 2 {
                  }
                }
                n3428 = for {
                  N: 32 -> [_]
                  tunnel: w5862 -> [w5887]
                  i -> [w5882]
                  # "①"
                  # "※複製コピーはこのケースで行う"
                  # "32回分"
                  # "比較する固定GNO"
                  n3429 = local read "メイン設定_設定 10"() -> (w5881:T2)
                  n3430 = Index Array(array=w5887, index=w5882) -> (element=w5886:T2)
                  n3431 = Unbundle By Name(w5881) -> ("ポートNo."=w5885:dbl)
                  n3432 = Unbundle By Name(w5886) -> ("ポートNo."=w5884:dbl)
                  n3433 = Equal?(x=w5885, y=w5884) -> (x = y?=w5883:bool)
                  n3434 = case shown="TRUE" w5883 {
                    tunnel: w5886 -> [_ w5888]
                    tunnel: w5882 -> [_ w5889]
                    frame False {
                    }
                    frame True {
                      n3435 = case shown="0, デフォルト" w5889 {
                        tunnel: w5888 -> [w5905 w5923 w5941 w5959 w5977 w5995 w6013 w6031 w6049 w6067 w6085 w6103]
                        tunnel: w5889 -> [w5904 w5922 w5940 w5958 w5976 w5994 w6012 w6030 w6048 w6066 w6084 w6102]
                        frame 0, Default {
                          w5895 = 2
                          # "B"
                          # "A"
                          # "csv作成の為表へクラスタ(実測値)書き込み"
                          # "⑤"
                          # "③"
                          # "④"
                          n3436 = local read "メインON/OFF_\n設定 1"() -> (w5906:T1)
                          n3437 = Unbundle By Name(w5906) -> ("使用ON/OFF"=w5902:bool)
                          n3438 = control-ref of="前回値転記用配列"() -> (w5900:refnum<vi>)
                          n3439 = local read "メイン設定_設定 1"() -> (w5907:T2)
                          n3440 = call "メイン_測定値配列_CSV転記サブ.vi"("メイン設定_設定入力"=w5907, "ループ反復数値入力"=w5904, "実測設定項目"=w5905, "使用ON/OFF"=w5902, "前回値転記用配列"=w5900) -> ("ループ反復数値出力"=w5903:i32, "メイン設定_設定出力"=w5901:T2)  [unwired: 5 in]
                          n3441 = local write "メイン設定_設定 1"(w5901) -> ()
                          n3442 = Add(x=2, y=w5903) -> (x+y=w5896:i32)
                          n3443 = Add(x=w5903, y=3) -> (x+y=w5894:i32)
                          n3444 = local read "csv作成表"() -> (w5890:string[][])
                          n3445 = Unbundle By Name(w5901) -> ("実測値(MAX)"=w5897:string, "実測値(MIN)"=w5898:string)
                          n3446 = Replace Array Subset(array=w5890, new element #1=w5897, index (row) #1=w5895, index (col) #1=w5896, new element #2=w5898, index (row) #2=w5895, index (col) #2=w5894) -> (w5892:string[][])
                          n3447 = Select(t=w5892, s=w5902, f=w5890) -> (s? t:f=w5893:string[][])
                          n3448 = local write "csv作成表"(w5893) -> ()
                        }
                        frame 1 {
                          w5913 = 2
                          # "B"
                          # "A"
                          # "csv作成の為表へクラスタ(実測値)書き込み"
                          # "⑤"
                          # "③"
                          # "④"
                          n3449 = local read "メインON/OFF_\n設定 2"() -> (w5924:T1)
                          n3450 = Unbundle By Name(w5924) -> ("使用ON/OFF"=w5920:bool)
                          n3451 = control-ref of="前回値転記用配列"() -> (w5918:refnum<vi>)
                          n3452 = local read "メイン設定_設定 2"() -> (w5925:T2)
                          n3453 = call "メイン_測定値配列_CSV転記サブ.vi"("メイン設定_設定入力"=w5925, "ループ反復数値入力"=w5922, "実測設定項目"=w5923, "使用ON/OFF"=w5920, "前回値転記用配列"=w5918) -> ("ループ反復数値出力"=w5921:i32, "メイン設定_設定出力"=w5919:T2)  [unwired: 5 in]
                          n3454 = local write "メイン設定_設定 2"(w5919) -> ()
                          n3455 = Add(x=3, y=w5921) -> (x+y=w5914:i32)
                          n3456 = Add(x=w5921, y=4) -> (x+y=w5912:i32)
                          n3457 = local read "csv作成表"() -> (w5908:string[][])
                          n3458 = Unbundle By Name(w5919) -> ("実測値(MAX)"=w5915:string, "実測値(MIN)"=w5916:string)
                          n3459 = Replace Array Subset(array=w5908, new element #1=w5915, index (row) #1=w5913, index (col) #1=w5914, new element #2=w5916, index (row) #2=w5913, index (col) #2=w5912) -> (w5910:string[][])
                          n3460 = Select(t=w5910, s=w5920, f=w5908) -> (s? t:f=w5911:string[][])
                          n3461 = local write "csv作成表"(w5911) -> ()
                        }
                        frame 2 {
                          w5931 = 2
                          # "B"
                          # "A"
                          # "csv作成の為表へクラスタ(実測値)書き込み"
                          # "⑤"
                          # "③"
                          # "④"
                          n3462 = local read "メインON/OFF_\n設定 3"() -> (w5942:T1)
                          n3463 = Unbundle By Name(w5942) -> ("使用ON/OFF"=w5938:bool)
                          n3464 = control-ref of="前回値転記用配列"() -> (w5936:refnum<vi>)
                          n3465 = local read "メイン設定_設定 3"() -> (w5943:T2)
                          n3466 = call "メイン_測定値配列_CSV転記サブ.vi"("メイン設定_設定入力"=w5943, "ループ反復数値入力"=w5940, "実測設定項目"=w5941, "使用ON/OFF"=w5938, "前回値転記用配列"=w5936) -> ("ループ反復数値出力"=w5939:i32, "メイン設定_設定出力"=w5937:T2)  [unwired: 5 in]
                          n3467 = local write "メイン設定_設定 3"(w5937) -> ()
                          n3468 = Add(x=4, y=w5939) -> (x+y=w5932:i32)
                          n3469 = Add(x=w5939, y=5) -> (x+y=w5930:i32)
                          n3470 = local read "csv作成表"() -> (w5926:string[][])
                          n3471 = Unbundle By Name(w5937) -> ("実測値(MAX)"=w5933:string, "実測値(MIN)"=w5934:string)
                          n3472 = Replace Array Subset(array=w5926, new element #1=w5933, index (row) #1=w5931, index (col) #1=w5932, new element #2=w5934, index (row) #2=w5931, index (col) #2=w5930) -> (w5928:string[][])
                          n3473 = Select(t=w5928, s=w5938, f=w5926) -> (s? t:f=w5929:string[][])
                          n3474 = local write "csv作成表"(w5929) -> ()
                        }
                        frame 3 {
                          w5949 = 2
                          # "B"
                          # "A"
                          # "csv作成の為表へクラスタ(実測値)書き込み"
                          # "⑤"
                          # "③"
                          # "④"
                          n3475 = local read "メインON/OFF_\n設定 4"() -> (w5960:T1)
                          n3476 = Unbundle By Name(w5960) -> ("使用ON/OFF"=w5956:bool)
                          n3477 = control-ref of="前回値転記用配列"() -> (w5954:refnum<vi>)
                          n3478 = local read "メイン設定_設定 4"() -> (w5961:T2)
                          n3479 = call "メイン_測定値配列_CSV転記サブ.vi"("メイン設定_設定入力"=w5961, "ループ反復数値入力"=w5958, "実測設定項目"=w5959, "使用ON/OFF"=w5956, "前回値転記用配列"=w5954) -> ("ループ反復数値出力"=w5957:i32, "メイン設定_設定出力"=w5955:T2)  [unwired: 5 in]
                          n3480 = local write "メイン設定_設定 4"(w5955) -> ()
                          n3481 = Add(x=5, y=w5957) -> (x+y=w5950:i32)
                          n3482 = Add(x=w5957, y=6) -> (x+y=w5948:i32)
                          n3483 = local read "csv作成表"() -> (w5944:string[][])
                          n3484 = Unbundle By Name(w5955) -> ("実測値(MAX)"=w5951:string, "実測値(MIN)"=w5952:string)
                          n3485 = Replace Array Subset(array=w5944, new element #1=w5951, index (row) #1=w5949, index (col) #1=w5950, new element #2=w5952, index (row) #2=w5949, index (col) #2=w5948) -> (w5946:string[][])
                          n3486 = Select(t=w5946, s=w5956, f=w5944) -> (s? t:f=w5947:string[][])
                          n3487 = local write "csv作成表"(w5947) -> ()
                        }
                        frame 4 {
                          w5967 = 2
                          # "B"
                          # "A"
                          # "csv作成の為表へクラスタ(実測値)書き込み"
                          # "⑤"
                          # "③"
                          # "④"
                          n3488 = local read "メインON/OFF_\n設定 5"() -> (w5978:T1)
                          n3489 = Unbundle By Name(w5978) -> ("使用ON/OFF"=w5974:bool)
                          n3490 = control-ref of="前回値転記用配列"() -> (w5972:refnum<vi>)
                          n3491 = local read "メイン設定_設定 5"() -> (w5979:T2)
                          n3492 = call "メイン_測定値配列_CSV転記サブ.vi"("メイン設定_設定入力"=w5979, "ループ反復数値入力"=w5976, "実測設定項目"=w5977, "使用ON/OFF"=w5974, "前回値転記用配列"=w5972) -> ("ループ反復数値出力"=w5975:i32, "メイン設定_設定出力"=w5973:T2)  [unwired: 5 in]
                          n3493 = local write "メイン設定_設定 5"(w5973) -> ()
                          n3494 = Add(x=6, y=w5975) -> (x+y=w5968:i32)
                          n3495 = Add(x=w5975, y=7) -> (x+y=w5966:i32)
                          n3496 = local read "csv作成表"() -> (w5962:string[][])
                          n3497 = Unbundle By Name(w5973) -> ("実測値(MAX)"=w5969:string, "実測値(MIN)"=w5970:string)
                          n3498 = Replace Array Subset(array=w5962, new element #1=w5969, index (row) #1=w5967, index (col) #1=w5968, new element #2=w5970, index (row) #2=w5967, index (col) #2=w5966) -> (w5964:string[][])
                          n3499 = Select(t=w5964, s=w5974, f=w5962) -> (s? t:f=w5965:string[][])
                          n3500 = local write "csv作成表"(w5965) -> ()
                        }
                        frame 5 {
                          w5985 = 2
                          # "B"
                          # "A"
                          # "csv作成の為表へクラスタ(実測値)書き込み"
                          # "⑤"
                          # "③"
                          # "④"
                          n3501 = local read "メインON/OFF_\n設定 6"() -> (w5996:T1)
                          n3502 = Unbundle By Name(w5996) -> ("使用ON/OFF"=w5992:bool)
                          n3503 = control-ref of="前回値転記用配列"() -> (w5990:refnum<vi>)
                          n3504 = local read "メイン設定_設定 6"() -> (w5997:T2)
                          n3505 = call "メイン_測定値配列_CSV転記サブ.vi"("メイン設定_設定入力"=w5997, "ループ反復数値入力"=w5994, "実測設定項目"=w5995, "使用ON/OFF"=w5992, "前回値転記用配列"=w5990) -> ("ループ反復数値出力"=w5993:i32, "メイン設定_設定出力"=w5991:T2)  [unwired: 5 in]
                          n3506 = local write "メイン設定_設定 6"(w5991) -> ()
                          n3507 = Add(x=7, y=w5993) -> (x+y=w5986:i32)
                          n3508 = Add(x=w5993, y=8) -> (x+y=w5984:i32)
                          n3509 = local read "csv作成表"() -> (w5980:string[][])
                          n3510 = Unbundle By Name(w5991) -> ("実測値(MAX)"=w5987:string, "実測値(MIN)"=w5988:string)
                          n3511 = Replace Array Subset(array=w5980, new element #1=w5987, index (row) #1=w5985, index (col) #1=w5986, new element #2=w5988, index (row) #2=w5985, index (col) #2=w5984) -> (w5982:string[][])
                          n3512 = Select(t=w5982, s=w5992, f=w5980) -> (s? t:f=w5983:string[][])
                          n3513 = local write "csv作成表"(w5983) -> ()
                        }
                        frame 6 {
                          w6003 = 2
                          # "B"
                          # "A"
